vi "FABR-Init Neural Plot.vi"(0 "XYGraph in":refnum<vi>, 5 "XAxis":refnum<vi>, 7 "YAxis":refnum<vi>, 9 "Freq":dbl[](array[numeric]), 11 "Level":dbl[](array[numeric])) -> (15 "error out":errorcluster)   [LabVIEW 2020]
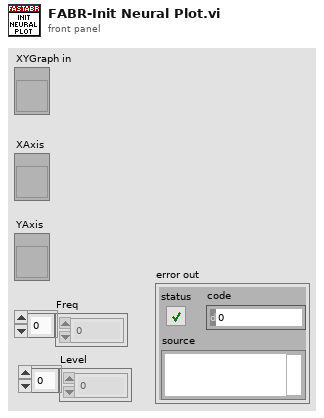
[diagram p1: front panel]
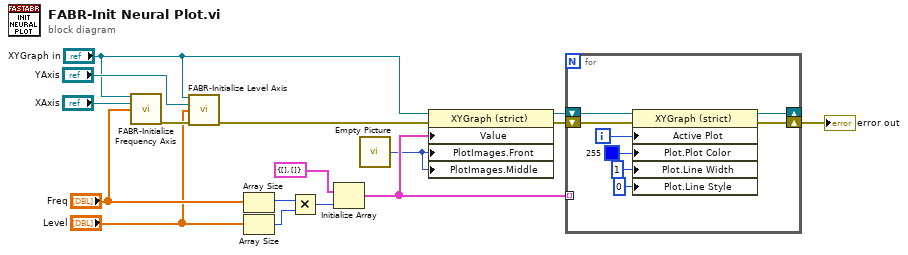
[diagram p0: block diagram]
diagram:
  n1 = call "FABR-Initialize Frequency Axis.vi"("XYGraph in"="XYGraph in", "FreqAxisLabel"="XAxis", "Array"="Freq") -> ("error out"=w15:errorcluster)  [unwired: 12 in]
  n2 = call "FABR-Initialize Level Axis.vi"("XYGraph in"="XYGraph in", "YAxis"="YAxis", "Levels"="Level", "error in (no error)"=w15) -> ("error out"=w10:errorcluster)  [unwired: 11 in]
  n3 = Array Size(array="Freq") -> (size(s)=w9:i32)
  n4 = Array Size(array="Level") -> (size(s)=w8:i32)
  n5 = Multiply(x=w9, y=w8) -> (x*y=w7:i32)
  n6 = Initialize Array(cluster{dbl[], dbl[]} {[], []}, w7) -> (w2:cluster{dbl[], dbl[]}[])
  n7 = call "Empty Picture"() -> ("empty picture"=w1:picture)
  n8 = property class="XYGraph (strict)"(reference="XYGraph in", error in=w10, "Value"=w2, "PlotImages.Front"=w1, "PlotImages.Middle"=w1) -> (reference out=w5:refnum<vi>, error out=w4:errorcluster)
  n9 = for {
    shift-right: [w18] -> _
    shift-left: w5 -> [w24]
    shift-right: [w17] -> w3
    shift-left: w4 -> [w23]
    tunnel: w2 -> [_] mode=indexing
    i -> [w22]
    n10 = property class="XYGraph (strict)"(reference=w24, error in=w23, "Active Plot"=w22, "Plot.Plot Color"=u32 255, "Plot.Line Width"=u8 1, "Plot.Line Style"=u8 0) -> (reference out=w18:refnum<vi>, error out=w17:errorcluster)
  }
  "error out" <- w3
